vi "Get - Time Data OBJ.vi"(0 "reference in":refnum<class "AdvSigProc.lvclass">, 5 "error in (no error)":errorcluster) -> (13 "New Time Data Obj?":bool, 14 "reference out":refnum<class "AdvSigProc.lvclass">, 16 "GSwFormDSP":refnum<class "GSwFormDSP.lvclass">, 19 "error out":errorcluster)   [LabVIEW 2020, in "AdvSigProc.lvclass"]
uses:
  AdvSigProc.lvclass
  API/GSwFormDSP_class/GSwFormDSP.lvclass
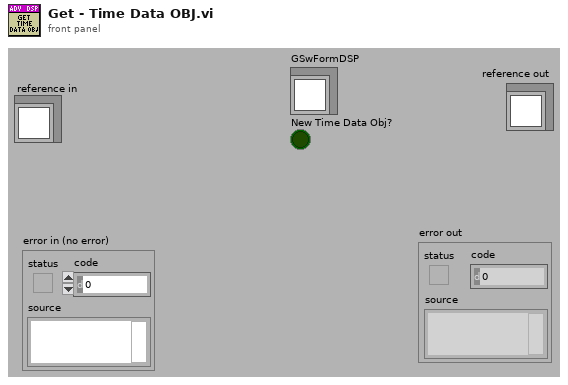
[diagram p1: front panel]
types:
  T1 = typedef "AdvSigProc.lvclass/ObjectAttributes.ctl" = cluster{"Time Data":cluster{"New Time Data Obj?":bool, "GSwFormDSP":refnum<class "GSwFormDSP.lvclass">}, "LMS Parameters":T2}
  T2 = typedef "AdvSigProc.lvclass/LMS.ctl" = cluster{"adaptive filter Ref":refnum<k20>, "Filtered Signals":refnum<class "GSwFormDSP.lvclass">, "Filter Coefs":dbl[], "Input Parameters":T3, "Iteration Metrics":T4[]}
  T3 = typedef "AdvSigProc.lvclass/LMS Input Parameters.ctl" = cluster{"Type":enum16{"Normalized LMS", "LMS", "FIR Sign LMS", "FIR Fast Block LMS", "RLS", "QR - RLS"}, "Filter Class":enum16{"Noise Cancelling (BGN Ref)", "Noise Cancelling (Speech Ref)"}, "Filter Length":i32, "µ Parameters":cluster{"Type":enum16{"User Input", "Auto µ"}, "step size":dbl}, "Iterations":cluster{"Current":i32, "Maximum":i32}}
  T4 = typedef "AdvSigProc.lvclass/Iteration Metrics.ctl" = cluster{"Name":string, "Max":dbl, "Min":dbl, "Values History":dbl[]}
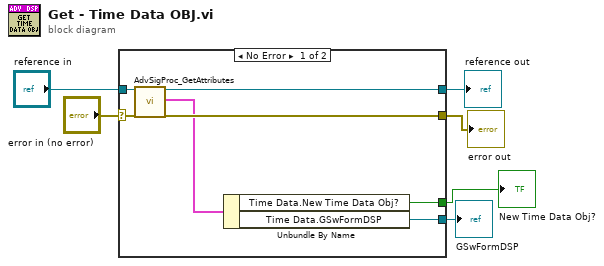
[diagram p0: block diagram]
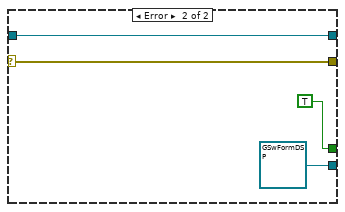
[diagram p2: hidden frame]
diagram:
  n1 = case shown="No Error" "error in (no error)" {
    selector: "error in (no error)" -> [w13 w17]
    tunnel: [w12 w17] -> w5
    tunnel: [w11 w16] -> w3
    tunnel: "reference in" -> [w9 w16]
    tunnel: [w8 refnum<class "GSwFormDSP.lvclass"> refnum ("GSwFormDSP")] -> w2
    tunnel: [w7 TRUE ("New Time Data Obj?")] -> w1
    frame No Error {
      n2 = call "AdvSigProc_GetAttributes.vi"("reference in"=w9, "error in (no error)"=w13) -> ("reference out"=w11:refnum<class "AdvSigProc.lvclass">, "attributes"=w10:T1, "error out"=w12:errorcluster)  [unwired: 14 in, 1 out]
      n3 = Unbundle By Name(w10) -> ("Time Data.New Time Data Obj?"=w7:bool, "Time Data.GSwFormDSP"=w8:refnum<class "GSwFormDSP.lvclass">)
    }
    frame Error {
    }
  }
  "error out" <- w5
  "reference out" <- w3
  "GSwFormDSP" <- w2
  "New Time Data Obj?" <- w1
